vi "Write Power-up Settings.vi"(7 "Unit ID (A)":string="A", 8 "error in":errorcluster, 10 "Power-up settings":T1={"Serial/Local Setpoint"=enum."Save", "Initial Screen"=enum."Main", "Gas Select"=enum."Save"}, 11 "VISA Session In":refnum<visa-resource-name>="Alicat") -> (0 "error out":errorcluster, 3 "VISA Session Out":refnum<visa-resource-name>)   [LabVIEW 2016]
doc: "Writes the options for the saving of serial/local setpoints, the initial screen option, and the selected gas to the EEPROM of an Alicat device.\n\nIF WRITING MULTIPLE SETPOINTS PER SECOND: DISABLE SAVING SERIAL/LOCAL SETPOINTS TO PREVENT BURNING OUT THE EEPROM OF THE ALICAT DEVICE."
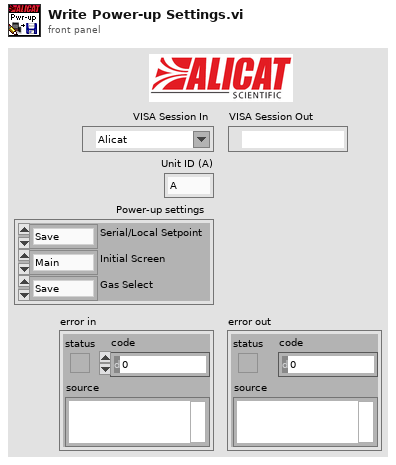
[diagram p1: front panel]
types:
  T1 = cluster{"Serial/Local Setpoint":enum8{"Don't Save", "Save"}, "Initial Screen":enum16{"Main", "Totalizer"}, "Gas Select":enum8{"Don't Save", "Save"}}
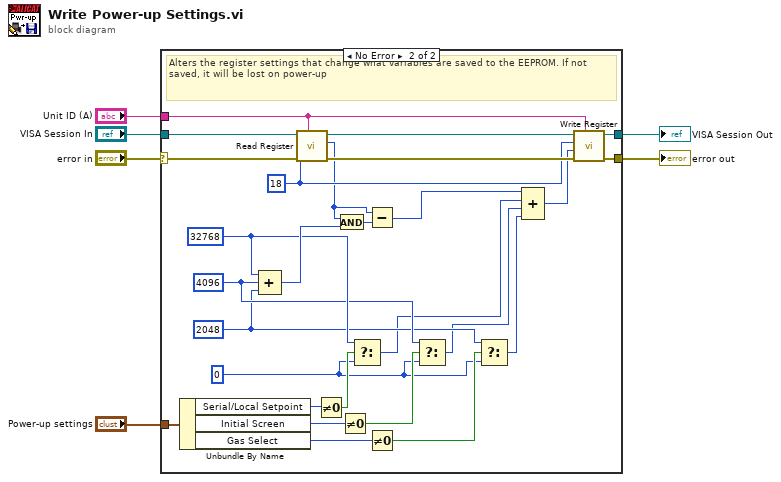
[diagram p0: block diagram]
diagram:
  n1 = case shown="No Error" "error in" {
    selector: "error in" -> [w7 w35]
    tunnel: "VISA Session In" -> [w8 w34]
    tunnel: [w7 w16] -> w4
    tunnel: [w8 w32] -> w3
    tunnel: "Unit ID (A)" -> [_ w30]
    tunnel: "Power-up settings" -> [_ w28]
    frame Error {
    }
    frame No Error {
      w20 = 0 ("y")
      w12 = 2048 ("y")
      w14 = 4096 ("y")
      w15 = 32768 ("y")
      w17 = u16 18 ("register")
      # "Alters the register settings that change what variables are saved to the EEPROM. If not saved, it will be lost on power-up"
      n2 = Unbundle By Name(w28) -> ("Serial/Local Setpoint"=w26:enum8{"Don't Save", "Save"}, "Initial Screen"=w25:enum16{"Main", "Totalizer"}, "Gas Select"=w24:enum8{"Don't Save", "Save"})
      n3 = Compound Arithmetic op=unknown(w15, w14, w12) -> (w29:i32)
      n4 = call "Read Register.vi"("Unit ID (A)"=w30, "error in"=w35, "Register address"=w17, "VISA Session In"=w34) -> ("error out"=w33:errorcluster, "Register Value (I32)"=w13:i32, "VISA Session Out"=w31:refnum<visa-resource-name>)  [unwired: 5 in]
      n5 = Not Equal To 0?(x=w26) -> (x != 0?=w21:bool)
      n6 = And(x=w13, y=w29) -> (x .and. y?=w27:i32)
      n7 = Not Equal To 0?(x=w25) -> (x != 0?=w22:bool)
      n8 = Select(t=w15, s=w21, f=w20) -> (s? t:f=w11:i32)
      n9 = Subtract(x=w13, y=w27) -> (x-y=w19:i32)
      n10 = Not Equal To 0?(x=w24) -> (x != 0?=w23:bool)
      n11 = Select(t=w14, s=w22, f=w20) -> (s? t:f=w10:i32)
      n12 = Select(t=w12, s=w23, f=w20) -> (s? t:f=w9:i32)
      n13 = Compound Arithmetic op=ADD(w19, w11, w10, w9) -> (w18:i32)
      n14 = call "Write Register.vi"("Unit ID (A)"=w30, "error in"=w33, "Register Value"=w18, "Register address"=w17, "VISA Session In"=w31) -> ("error out"=w16:errorcluster, "VISA Session Out"=w32:refnum<visa-resource-name>)  [unwired: 4 in, 1 out]
    }
  }
  "error out" <- w4
  "VISA Session Out" <- w3
